vi "Preprocess_and_Convert_IMAQ_Image_to_Array.vi"(7 "PreProcessing_Options":T2={"DS_Name"="delete", "Input_Dims"={"C"=3, "H"=224, "W"=224}, "Center Crop Size"=0, "Interpolation Type"=1, "Multi-Stage_DownSample?"=FALSE, "Dataset_Stats"={"means"={"R"=0.5385, "G"=0.5348, "B"=0.551}, "stds"={"R"=0.3673, "G"=0.3673, "B"=0.3505}}} {"Dataset_Stats"."stds"."R" format="%#_3g"; "Dataset_Stats"."stds"."G" format="%#_3g"; "Dataset_Stats"."stds"."B" format="%#_3g"; "Dataset_Stats"."means"."R" format="%#_3g"; "Dataset_Stats"."means"."G" format="%#_3g"; "Dataset_Stats"."means"."B" format="%#_3g"; "Interpolation Type" items=["Zero Order", "Bi-Linear", "Quadratic", "Cubic Spline"]}, 8 "error in (no error)":errorcluster, 11 "Imaq Image In":T1=refnum) -> (0 "error out":errorcluster, 2 "Norm_Img_Out":sgl[][][](array[numeric]), 3 "Imaq Image Out":T1, 5 "dT_Preprocessing":dbl=0.0017125000013038516)   [LabVIEW 2020]
uses:
  <vilib>/Ngene/DeepLTK Anomaly Detection Addon/DeepLTK_Anomaly_Detection_Addon/API/Controls/NNPC_PreProcessing_Options.ctl
  <vilib>/Ngene/Deep Learning Toolkit/Toolkit/NN_Data/API/NN_Dims(C,H,W).ctl
  <vilib>/Ngene/DeepLTK Anomaly Detection Addon/DeepLTK_Anomaly_Detection_Addon/API/Controls/NNPC_DS_Stats.ctl
  <vilib>/Ngene/DeepLTK Anomaly Detection Addon/DeepLTK_Anomaly_Detection_Addon/API/Controls/Image_Stats_RGB.ctl
  <vilib>/vision/Image Controls.llb/IMAQ Image.ctl
  <vilib>/vision/NI_Vision_Development_Module.lvlib
  <vilib>/Ngene/Deep Learning Toolkit/Toolkit/Deep_Learning_Toolkit_by_Ngene.lvlib
  <vilib>/Ngene/DeepLTK Anomaly Detection Addon/DeepLTK_Anomaly_Detection_Addon/DeepLTK_Anomaly_Detection_Addon.lvlib
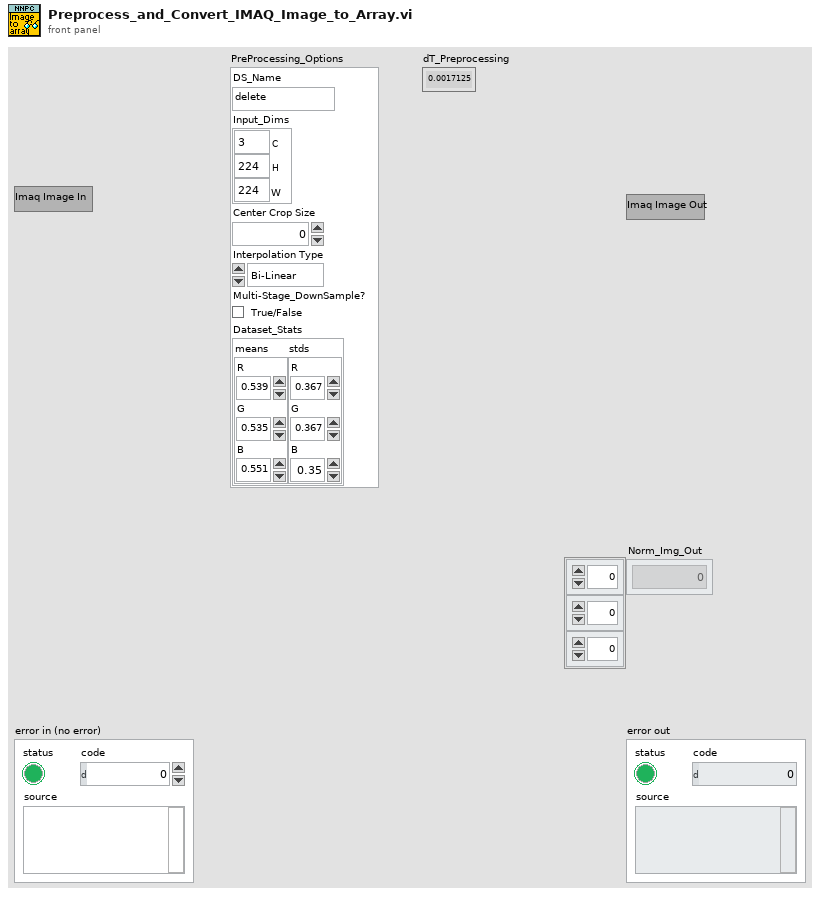
[diagram p1: front panel]
types:
  T1 = typedef "IMAQ Image.ctl" = refnum<image>
  T2 = typedef "DeepLTK_Anomaly_Detection_Addon.lvlib/NNPC_PreProcessing_Options.ctl" = cluster{"DS_Name":string, "Input_Dims":T3, "Center Crop Size":i32, "Interpolation Type":u32, "Multi-Stage_DownSample?":bool, "Dataset_Stats":T4}
  T3 = typedef "Deep_Learning_Toolkit_by_Ngene.lvlib/NN_Dims(C,H,W).ctl" = cluster{"C":i32, "H":i32, "W":i32}
  T4 = typedef "DeepLTK_Anomaly_Detection_Addon.lvlib/NNPC_DS_Stats.ctl" = cluster{"means":T5, "stds":T5}
  T5 = typedef "DeepLTK_Anomaly_Detection_Addon.lvlib/Image_Stats_RGB.ctl" = cluster{"R":sgl, "G":sgl, "B":sgl}
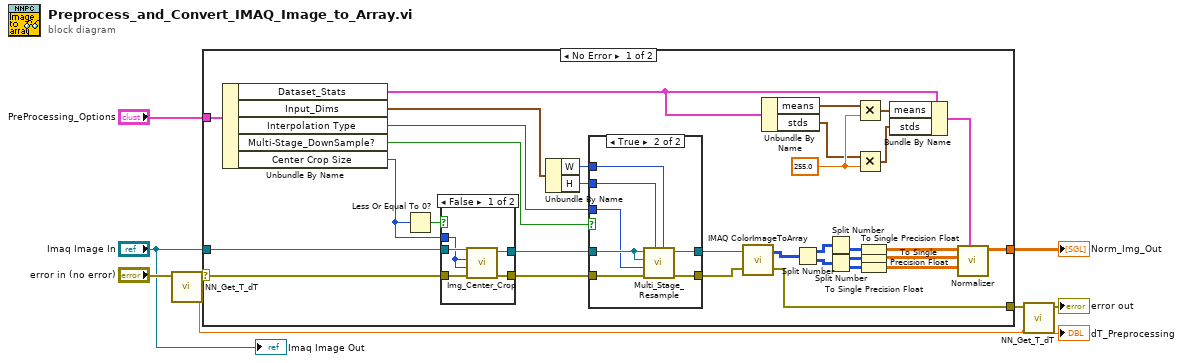
[diagram p0: block diagram]
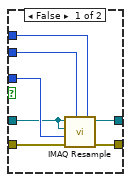
[diagram p2: hidden frame]
diagram:
  n1 = call <vilib>:"NN_Get_T_dT.vi"("error in (no error)"="error in (no error)") -> ("T_out"=w2:dbl, "error out"=w3:errorcluster)  [unwired: 6 in, 1 out]
  n2 = case shown="No Error" w3 {
    selector: w3 -> [w17 w63]
    tunnel: "PreProcessing_Options" -> [w41 _]
    tunnel: "Imaq Image In" -> [w16 _]
    tunnel: [w19 w63] -> w8
    tunnel: [w18 _] -> w7
    frame No Error {
      w33 = sgl 255.0 ("R")
      n3 = Unbundle By Name(w41) -> ("Dataset_Stats"=w34:T4, "Input_Dims"=w24:T3, "Interpolation Type"=w11:u32, "Multi-Stage_DownSample?"=w10:bool, "Center Crop Size"=w12:i32)
      n4 = Less Or Equal To 0?(x=w12) -> (x <= 0?=w13:bool)
      n5 = case shown="False" w13 {
        tunnel: w16 -> [w60 w62]
        tunnel: [w59 w62] -> w15
        tunnel: w17 -> [w58 w61]
        tunnel: [w57 w61] -> w14
        tunnel: w12 -> [w56 _]
        frame False {
          n6 = call "Img_Center_Crop.vi"("error in (no error)"=w58, "height"=w56, "width"=w56, "Image In"=w60) -> ("error out"=w57:errorcluster, "Image Out"=w59:T1)  [unwired: 6 in]
        }
        frame True {
        }
      }
      n7 = Unbundle By Name(w24) -> ("W"=w22:i32, "H"=w21:i32)
      n8 = case shown="True" w10 {
        tunnel: [w48 w52] -> w23
        tunnel: [w47 w53] -> w20
        tunnel: w11 -> [w46 w49]
        tunnel: w15 -> [w42 w50]
        tunnel: w22 -> [w45 w51]
        tunnel: w21 -> [w44 w54]
        tunnel: w14 -> [w43 w55]
        frame False {
          n9 = call "IMAQ Resample"("X Resolution"=w45, "Y Resolution"=w44, "error in (no error)"=w43, "Interpolation Type"=w46, "Image Dst"=w42, "Image Src"=w42) -> ("error out"=w48:errorcluster, "Image Dst Out"=w47:T1)  [unwired: 4 in]
        }
        frame True {
          n10 = call "Multi_Stage_Resample.vi"("X Resolution"=w51, "Y Resolution"=w54, "error in (no error)"=w55, "Interpolation Type"=w49, "Img in"=w50, "Dest"=w50) -> ("error out"=w52:errorcluster, "Img out"=w53:T1)  [unwired: 4 in]
        }
      }
      n11 = call "IMAQ ColorImageToArray"("Image"=w20, "error in (no error)"=w23) -> ("Image Pixels (U32)"=w30:u32[][], "error out"=w19:errorcluster)  [unwired: 2 in, 1 out]
      n12 = Unbundle By Name(w34) -> ("means"=w31:T5, "stds"=w32:T5)
      n13 = Split Number(x=w30) -> (hi(x)=w26:u16[][], lo(x)=w25:u16[][])
      n14 = Split Number(x=w26) -> (lo(x)=w27:u8[][])  [unwired: 1 out]
      n15 = Split Number(x=w25) -> (hi(x)=w28:u8[][], lo(x)=w29:u8[][])
      n16 = Multiply(x=w31, y=w33) -> (x*y=w36:T5)
      n17 = Multiply(x=w32, y=w33) -> (x*y=w37:T5)
      n18 = To Single Precision Float(number=w27) -> (single precision float=w38:sgl[][])
      n19 = To Single Precision Float(number=w28) -> (single precision float=w39:sgl[][])
      n20 = To Single Precision Float(number=w29) -> (single precision float=w40:sgl[][])
      n21 = Bundle By Name(cluster=w34, "means"=w36, "stds"=w37) -> (w35:T4)
      n22 = call "Normalizer.vi"("Dataset_Stats"=w35, "B"=w40, "G"=w39, "R"=w38) -> ("Norm_Img_Out"=w18:sgl[][][])  [unwired: 7 in]
    }
    frame Error {
    }
  }
  "Norm_Img_Out" <- w7
  n23 = call <vilib>:"NN_Get_T_dT.vi"("T_in"=w2, "error in (no error)"=w8) -> ("error out"=→"error out":errorcluster, "dT"=→"dT_Preprocessing":dbl)  [unwired: 5 in, 1 out]
  "Imaq Image Out" <- "Imaq Image In"
